vi "synnax client close.vi"(8 "error in":errorcluster, 11 "client":u64) -> (0 "error out":errorcluster)   [LabVIEW 2026, in "synnax_clib.lvlib"]
doc: "SYNNAX_EXPORT void synnax_client_close(SynnaxClient client);"
uses:
  synnax_clib.lvlib
  synnax_clib.dll
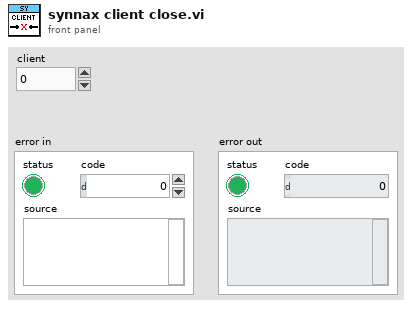
[diagram p1: front panel]
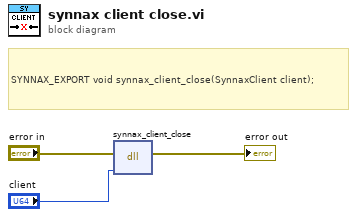
[diagram p0: block diagram]
diagram:
  # "SYNNAX_EXPORT void synnax_client_close(SynnaxClient client);"
  n1 = dll-call lib="C/synnax/client/labview/synnax_clib.dll" fn="synnax_client_close"(error in="error in", "client"="client") -> (error out=→"error out":errorcluster)  [unwired: 4 in, 1 out]
